vi "squarerootcalc.vi"() -> ()   [LabVIEW 2022 SP3]
uses:
  <vilib>/numeric/Random Number (Range) I64.vi
  <vilib>/numeric/sub_Random U32.vi
panel:
  in  "square root calc on/off":bool
  out "Rand number":dbl
  out "square root":dbl
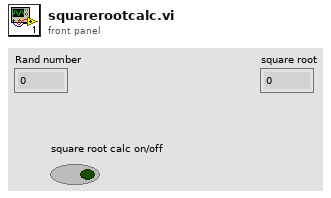
[diagram p1: front panel]
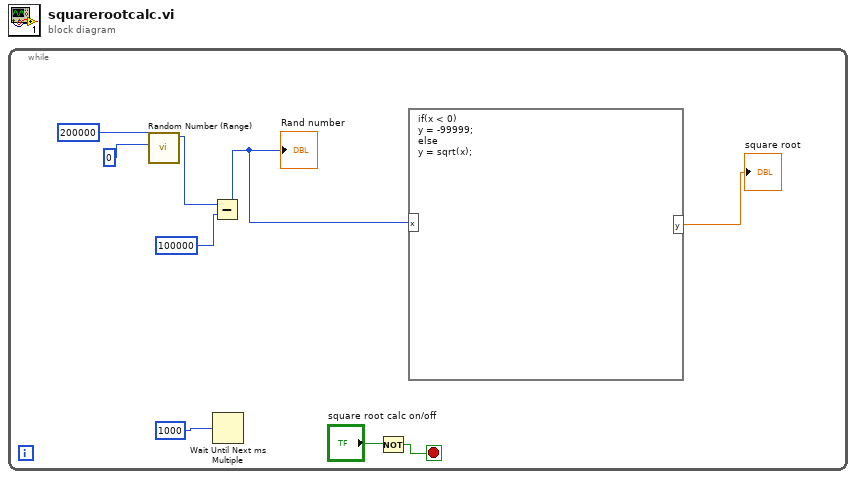
[diagram p0: block diagram]
diagram:
  n1 = while {
    stop <- w3 stop-if-true
    n2 = call-poly <vilib>:"Random Number (Range).vi"("lower bound (-100)"=0, "upper bound (100)"=200000) -> ("number"=w8:i64)  [unwired: 9 in]
    n3 = Subtract(x=w8, y=100000) -> (x-y=w2:i64)
    "Rand number" <- w2
    n4 = Wait Until Next ms Multiple(millisecond multiple=1000) -> ()  [unwired: 1 out]
    n5 = Not(x="square root calc on/off") -> (.not. x?=w3:bool)
    n6 = formula code="if(x < 0) \ny = -99999;\nelse\ny = sqrt(x);"("x"=w2) -> ("y"=→"square root":dbl)
  }
